vi "Resize Picture.vi"(0 "Picture ref":refnum<vi>, 5 "new width":i16, 7 "new height":i16) -> ()   [LabVIEW 2015, in "HRTF Config.xctl"]
uses:
  HRTF Config.xctl
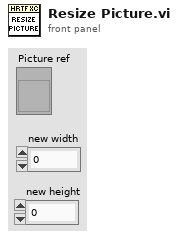
[diagram p1: front panel]
types:
  T1 = typedef "LVBoundsTypeDef.ctl" = cluster{"Width":u32, "Height":u32}
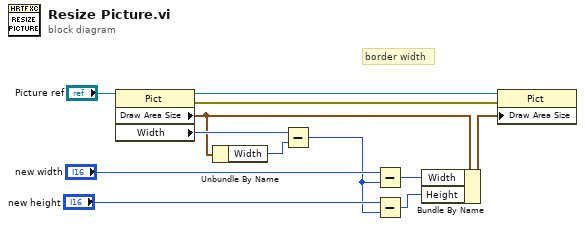
[diagram p0: block diagram]
diagram:
  # "border width"
  n1 = property class="Pict"(reference="Picture ref") -> (reference out=w6:refnum<vi>, error out=w7:errorcluster, "Draw Area Size"=w9:T1, "Width"=w10:u32)  [unwired: 1 in]
  n2 = Unbundle By Name(w9) -> ("Width"=w11:u32)
  n3 = Subtract(x=w10, y=w11) -> (x-y=w1:u32)
  n4 = Subtract(x="new width", y=w1) -> (x-y=w12:u32)
  n5 = Subtract(x="new height", y=w1) -> (x-y=w2:u32)
  n6 = Bundle By Name(cluster=w9, "Width"=w12, "Height"=w2) -> (w8:T1)
  n7 = property class="Pict"(reference=w6, error in=w7, "Draw Area Size"=w8) -> ()  [unwired: 2 out]
